vi "degreesToSteps.vi"(9 "theta3":dbl, 10 "theta2":dbl, 11 "theta1":dbl) -> (1 "steps3":dbl, 2 "steps2":dbl, 3 "steps1":dbl)   [LabVIEW 2020]
uses:
  globalVariable.vi
panel:
  out "theta3CP":dbl=-78.5639
  out "theta2CP":dbl=-78.5639
  out "theta1CP":dbl=-78.5639
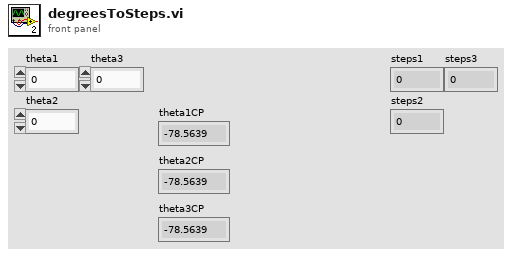
[diagram p1: front panel]
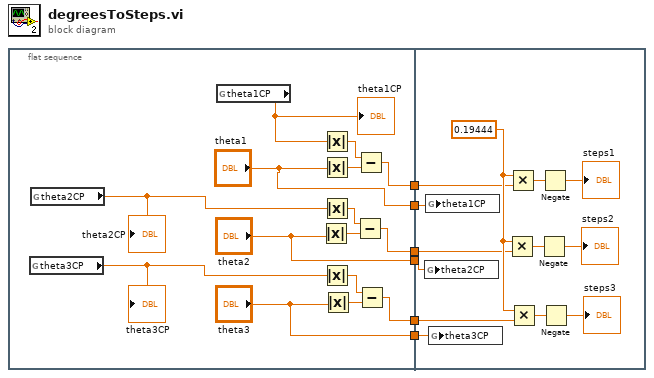
[diagram p0: block diagram]
diagram:
  n1 = flat-sequence {
    tunnel: [w15] -> w6
    tunnel: [w14] -> w5
    tunnel: [w13] -> w4
    tunnel: ["theta1"] -> w3
    tunnel: ["theta3"] -> w2
    tunnel: ["theta2"] -> w1
    tunnel: w6 -> [w25]
    tunnel: w5 -> [w27]
    tunnel: w4 -> [w26]
    tunnel: w3 -> [w24]
    tunnel: w2 -> [w23]
    tunnel: w1 -> [w22]
    frame #0 {
      n2 = global read "globalVariable.vi" "theta3CP"() -> (w9:dbl)
      "theta3CP" <- w9
      n3 = global read "globalVariable.vi" "theta2CP"() -> (w10:dbl)
      "theta2CP" <- w10
      n4 = global read "globalVariable.vi" "theta1CP"() -> (w11:dbl)
      "theta1CP" <- w11
      n5 = Absolute Value(x="theta2") -> (abs(x)=w18:dbl)
      n6 = Absolute Value(x=w11) -> (abs(x)=w19:dbl)
      n7 = Absolute Value(x="theta1") -> (abs(x)=w17:dbl)
      n8 = Absolute Value(x=w10) -> (abs(x)=w20:dbl)
      n9 = Absolute Value(x=w9) -> (abs(x)=w21:dbl)
      n10 = Absolute Value(x="theta3") -> (abs(x)=w16:dbl)
      n11 = Subtract(x=w20, y=w18) -> (x-y=w14:dbl)
      n12 = Subtract(x=w19, y=w17) -> (x-y=w15:dbl)
      n13 = Subtract(x=w21, y=w16) -> (x-y=w13:dbl)
    }
    frame #1 {
      w28 = 0.19444 ("x")
      n14 = global write "globalVariable.vi" "theta2CP"(w22) -> ()
      n15 = global write "globalVariable.vi" "theta1CP"(w24) -> ()
      n16 = global write "globalVariable.vi" "theta3CP"(w23) -> ()
      n17 = Multiply(x=w28, y=w27) -> (x*y=w32:dbl)
      n18 = Multiply(x=w28, y=w25) -> (x*y=w33:dbl)
      n19 = Multiply(x=w28, y=w26) -> (x*y=w34:dbl)
      n20 = Negate(x=w32) -> (-x=→"steps2":dbl)
      n21 = Negate(x=w33) -> (-x=→"steps1":dbl)
      n22 = Negate(x=w34) -> (-x=→"steps3":dbl)
    }
  }
